vi "closeNotifiers.vi"(8 "error in":errorcluster, 11 "notifiers":T1) -> (0 "error out":errorcluster)   [LabVIEW 2017, in "notifiers.lvlib"]
uses:
  notifiers.lvlib
  notifiers.ctl
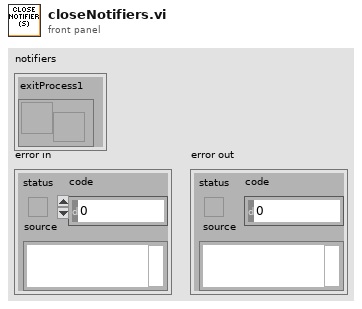
[diagram p1: front panel]
types:
  T1 = typedef "notifiers.lvlib/notifiers.ctl" = cluster{"exitProcess1":refnum<notifier>}
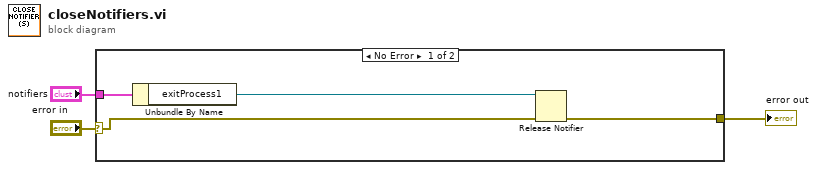
[diagram p0: block diagram]
diagram:
  n1 = case shown="No Error" "error in" {
    selector: "error in" -> [w4 w8]
    tunnel: "notifiers" -> [w7 _]
    tunnel: [w5 w8] -> w2
    frame No Error {
      n2 = Unbundle By Name(w7) -> ("exitProcess1"=w6:refnum<notifier>)
      n3 = Release Notifier(notifier=w6, error in (no error)=w4) -> (error out=w5:errorcluster)  [unwired: 1 in, 2 out]
    }
    frame Error {
    }
  }
  "error out" <- w2
